vi "Circulo.vi"() -> ()   [LabVIEW 2020]
panel:
  out "XY Grafico circulo":cluster{dbl[], dbl[]}(graph)
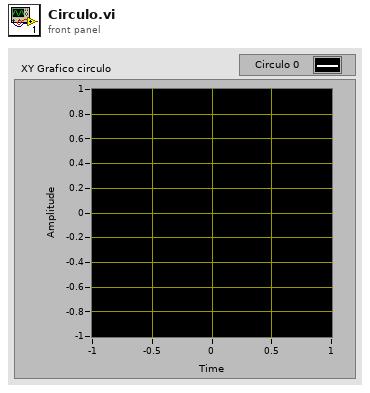
[diagram p1: front panel]
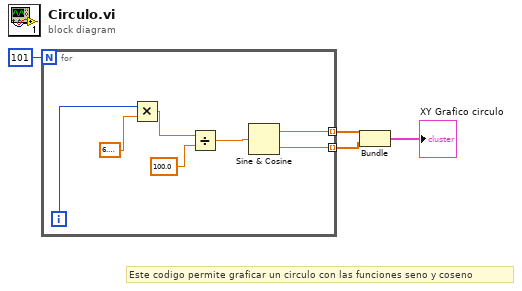
[diagram p0: block diagram]
diagram:
  # "Este codigo permite graficar un circulo con las funciones seno y coseno"
  n1 = for {
    N: 101 -> [_]
    tunnel: [w6] -> w3 mode=indexing
    tunnel: [w5] -> w2 mode=indexing
    i -> [w10]
    n2 = Multiply(x=w10, y=6.283185307179586) -> (x*y=w9:dbl)
    n3 = Divide(x=w9, y=100.0 ("x/y")) -> (x/y=w7:dbl)
    n4 = Sine & Cosine(0:w7) -> (1:w6:dbl, 2:w5:dbl)
  }
  n5 = Bundle(w3, w2) -> (→"XY Grafico circulo":cluster{dbl[], dbl[]})  [unwired: 1 in]
